vi "enumerateStaticDependencies.vi"(8 "error in (no error)":errorcluster, 11 "Microscope":refnum<class "Microscope.lvclass">) -> (0 "error out":errorcluster, 2 "Static Dependencies":refnum<class "Dependency.lvclass">[](array[class]), 3 "Microscope out":refnum<class "Microscope.lvclass">)   [LabVIEW 2013, in "Microscope.lvclass"]
doc: "JKI State Machine Objects (SMO) 1.1.0.20\nJKI - JKI\nCopyright (c) 2016, JKI"
uses:
  Microscope.lvclass
  <vilib>/JKI/JKI SMO/Dependency/Dependency.lvclass
  Camera/Camera.lvclass
  XYStage/XYStage.lvclass
  <vilib>/JKI/JKI SMO/SMO/SMO.lvclass
panel:
  # "For instructions on how to use the JKI State Machine Objects, examples and video tutorials, visit:\nhttp://jki.net/state-machine-objects/\n\nJKI State Machine Objects™\nhttp://jki.net/state-machine-objects/\nCopyright (C) 2005-2015, JKI <info@jki.net>\nALL RIGHTS RESERVED"
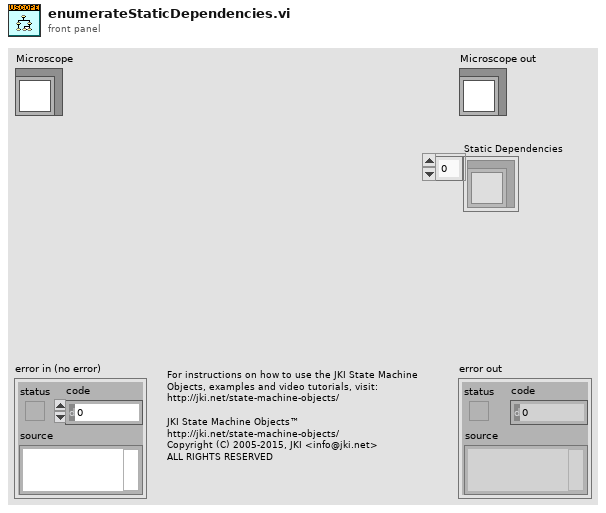
[diagram p1: front panel]
types:
  T1 = typedef "Microscope.lvclass/Configuration--Cluster.ctl" = cluster{"XY Stage":string, "Camera":string, "image output folder":path, "filetype":string}
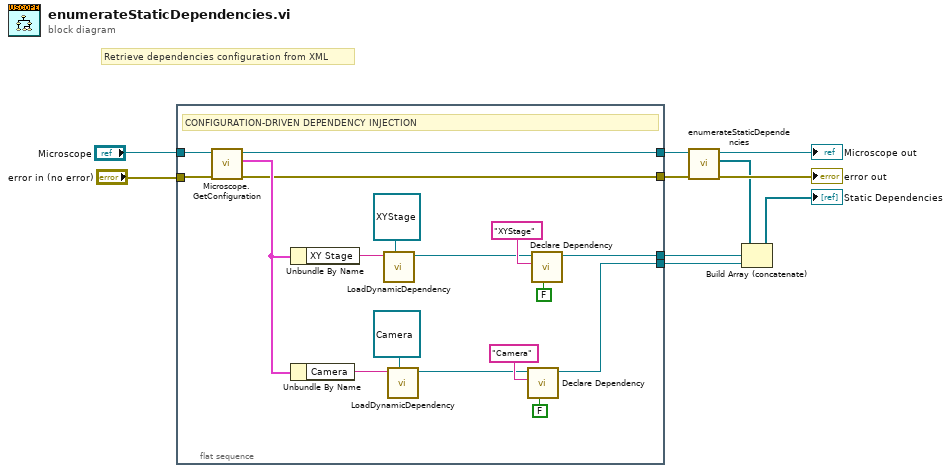
[diagram p0: block diagram]
diagram:
  # "Retrieve dependencies configuration from XML"
  n1 = flat-sequence {
    tunnel: "error in (no error)" -> [w21]
    tunnel: [w26] -> w5
    tunnel: [w20] -> w4
    tunnel: "Microscope" -> [w19]
    tunnel: [w12] -> w2
    tunnel: [w11] -> w1
    frame #0 {
      # "CONFIGURATION-DRIVEN DEPENDENCY INJECTION"
      n2 = call "Microscope.GetConfiguration.vi"("error in (no error)"=w21, "Microscope"=w19) -> ("error out"=w20:errorcluster, "Configuration"=w27:T1, "Microscope out"=w26:refnum<class "Microscope.lvclass">)  [unwired: 7 in]
      n3 = Unbundle By Name(w27) -> ("XY Stage"=w22:string)
      n4 = Unbundle By Name(w27) -> ("Camera"=w25:string)
      n5 = call "LoadDynamicDependency.vi"("SMO in"=refnum<class "XYStage.lvclass"> refnum ("XYStage.lvclass"), "Camera"=w22) -> ("SMO out"=w16:refnum<class "XYStage.lvclass">)  [unwired: 8 in, 1 out]
      n6 = call "LoadDynamicDependency.vi"("SMO in"=refnum<class "Camera.lvclass"> refnum ("Camera.lvclass"), "Camera"=w25) -> ("SMO out"=w13:refnum<class "Camera.lvclass">)  [unwired: 8 in, 1 out]
      n7 = call <vilib>:"Declare Dependency.vi"("Shared Resource (F)"=FALSE, "Name"="Camera", "Type"=w13) -> ("Dependency out"=w11:refnum<class "Dependency.lvclass">)  [unwired: 7 in, 1 out]
      n8 = call <vilib>:"Declare Dependency.vi"("Shared Resource (F)"=FALSE, "Name"="XYStage", "Type"=w16) -> ("Dependency out"=w12:refnum<class "Dependency.lvclass">)  [unwired: 7 in, 1 out]
    }
  }
  n9 = call-parent "enumerateStaticDependencies.vi"("error in (no error)"=w4, "SMO"=w5) -> ("error out"=→"error out":errorcluster, "Static Dependencies"=w7:refnum<class "Dependency.lvclass">[], "SMO out"=→"Microscope out":refnum<class "Microscope.lvclass">)  [unwired: 7 in]
  n10 = Build Array (concatenate)(w7, w2, w1) -> (→"Static Dependencies":refnum<class "Dependency.lvclass">[])
